vi "WildBugChilGru_V1.0.3.vi"() -> ()   [LabVIEW 2014]
uses:
  <vilib>/Utility/miscctls.llb/LVPointTypeDef.ctl
  <vilib>/Utility/xml.llb/Read From XML File(string).vi
  <vilib>/Utility/xml.llb/Write to XML File(string).vi
  <vilib>/gmath/NI_Gmath.lvlib
  <vilib>/Analysis/NI_AALBase.lvlib
  <vilib>/Analysis/NI_AALPro.lvlib
  <vilib>/Analysis/3filter.llb/IIR Filter (DBL).vi
  <vilib>/Instr/_visa.llb/VISA Configure Serial Port (Instr).vi
panel:
  in  "Registerkarte":T1(tab)
  in  "Zündung [Imp/U]":dbl=1.0
  in  "Übersetzung ermitteln aus":T2(ring)
  in  "Getriebe [1:]":dbl=5.343
  in  "Reifenumfang [m]":dbl=1.222
  in  "Dauer [s]":dbl=5.0
  in  "nKuWe/nRolle":dbl=10.0
  in  "Lufttemperatur [°C]":dbl=20.0
  in  "Luftfeuchtigkeit [%]":dbl=50.0
  in  "Luftdruck [mbar]":dbl=1013.0
  in  "Messung Klimadaten":bool=TRUE
  in  "Gleitender Mittelwert":u8=35
  in  "Differenzenquotient":u8=12
  in  "Polynom":u8=15
  in  "n vom Gas [1/min]":dbl=5000.0
  in  "Rollengeber [Inkr/U]":u16=200
  in  "Rollenumfang [m]":dbl=0.613
  in  "Rollenträgheit [kgm²]":dbl=0.402
  in  "Recalc":bool
  in  "Ende":bool
  out "Datenspeicher":T3={"Fahrzeugdaten"="", "date/time string"="", "Rolle [Inkr/U]"=0, "Rollenumfang [m]"=0.0, "Rollenträgheit [kgm²]"=0.0, "Zündung [Imp/U]"=0.0, "Getriebe [1:]"=0.0, "Reifenumfang [m] "=0.0, "element"=0.0, "Gl. Mittelwert"=0, "Differenzenquotient"=0, "Polynom"=0, "element"=0.0, "element"=0.0, "Lufttemperatur [°C]"=0.0, "Luftfeuchtigkeit [%]"=0.0, "Luftdruck [mbar]"=0.0, [], [], "Best Polynomial Fit"=[], [], "Übersetzung ermitteln aus"=0, "[s]"=0.0, "nmin [1/min]"=0.0, "nmax [1/min]"=0.0, "n vom Gas [1/min]"=0.0, [], [], "Boolesch"=FALSE, "Serielle Schnittstelle"="COM4", "nKuWe/nRolle"=10.0}
  out "COM-Fehlerrate":string="0 / 0,0%"
  in  "Konfiguration:":bool
  in  "Speichern":bool
  in  "Drucken":bool
  out "Pmax":string="0,0 PS"
  out "Ergebnis":string="0,0 PS bei 0 1/min   |   0,0 Nm bei 0 1/min   |   vmax: 2147483647 km/h\nDIN 70020 k =1,000 (20 °C, 50 %, 1013 mbar)\n20.11.2016 20:05 "
  in  "Fahrzeugdaten":string="Hier die Fahrzeugdaten eingeben"
  out "XY-Graph":cluster{dbl[], dbl[]}[](graph)
  out "Untersetzung\nermittelt":bool
  out "Untersetzung":dbl format="%#.2f"
  in  "Start":bool
  out "Füllstand Lesepuffer":u64(slide) scale=1.0..100.0
  out "Hinterrad\n[km/h]":dbl(knob) scale=0.0..150.0
  out "Welle\n[1/min]":cluster{dbl, dbl}(knob) scale=0.0..12000.0
  out "Lesepuffer":string="\n"
  in  "Serielle Schnittstelle":refnum<visa-resource-name>="COM4"
  out "Untersetzung-Graph":dbl(graph)=2.6802446808510636 caption="Untersetzung"
  # "1. n konstant halten\n2. START\n3. n weiter halten\n4. bei GO: Vollgas\n5. vom Gas gehen"
  # "Zündung\nRolle"
  # "Untersetzung aus:"
  # "Eingabe <> Messen"
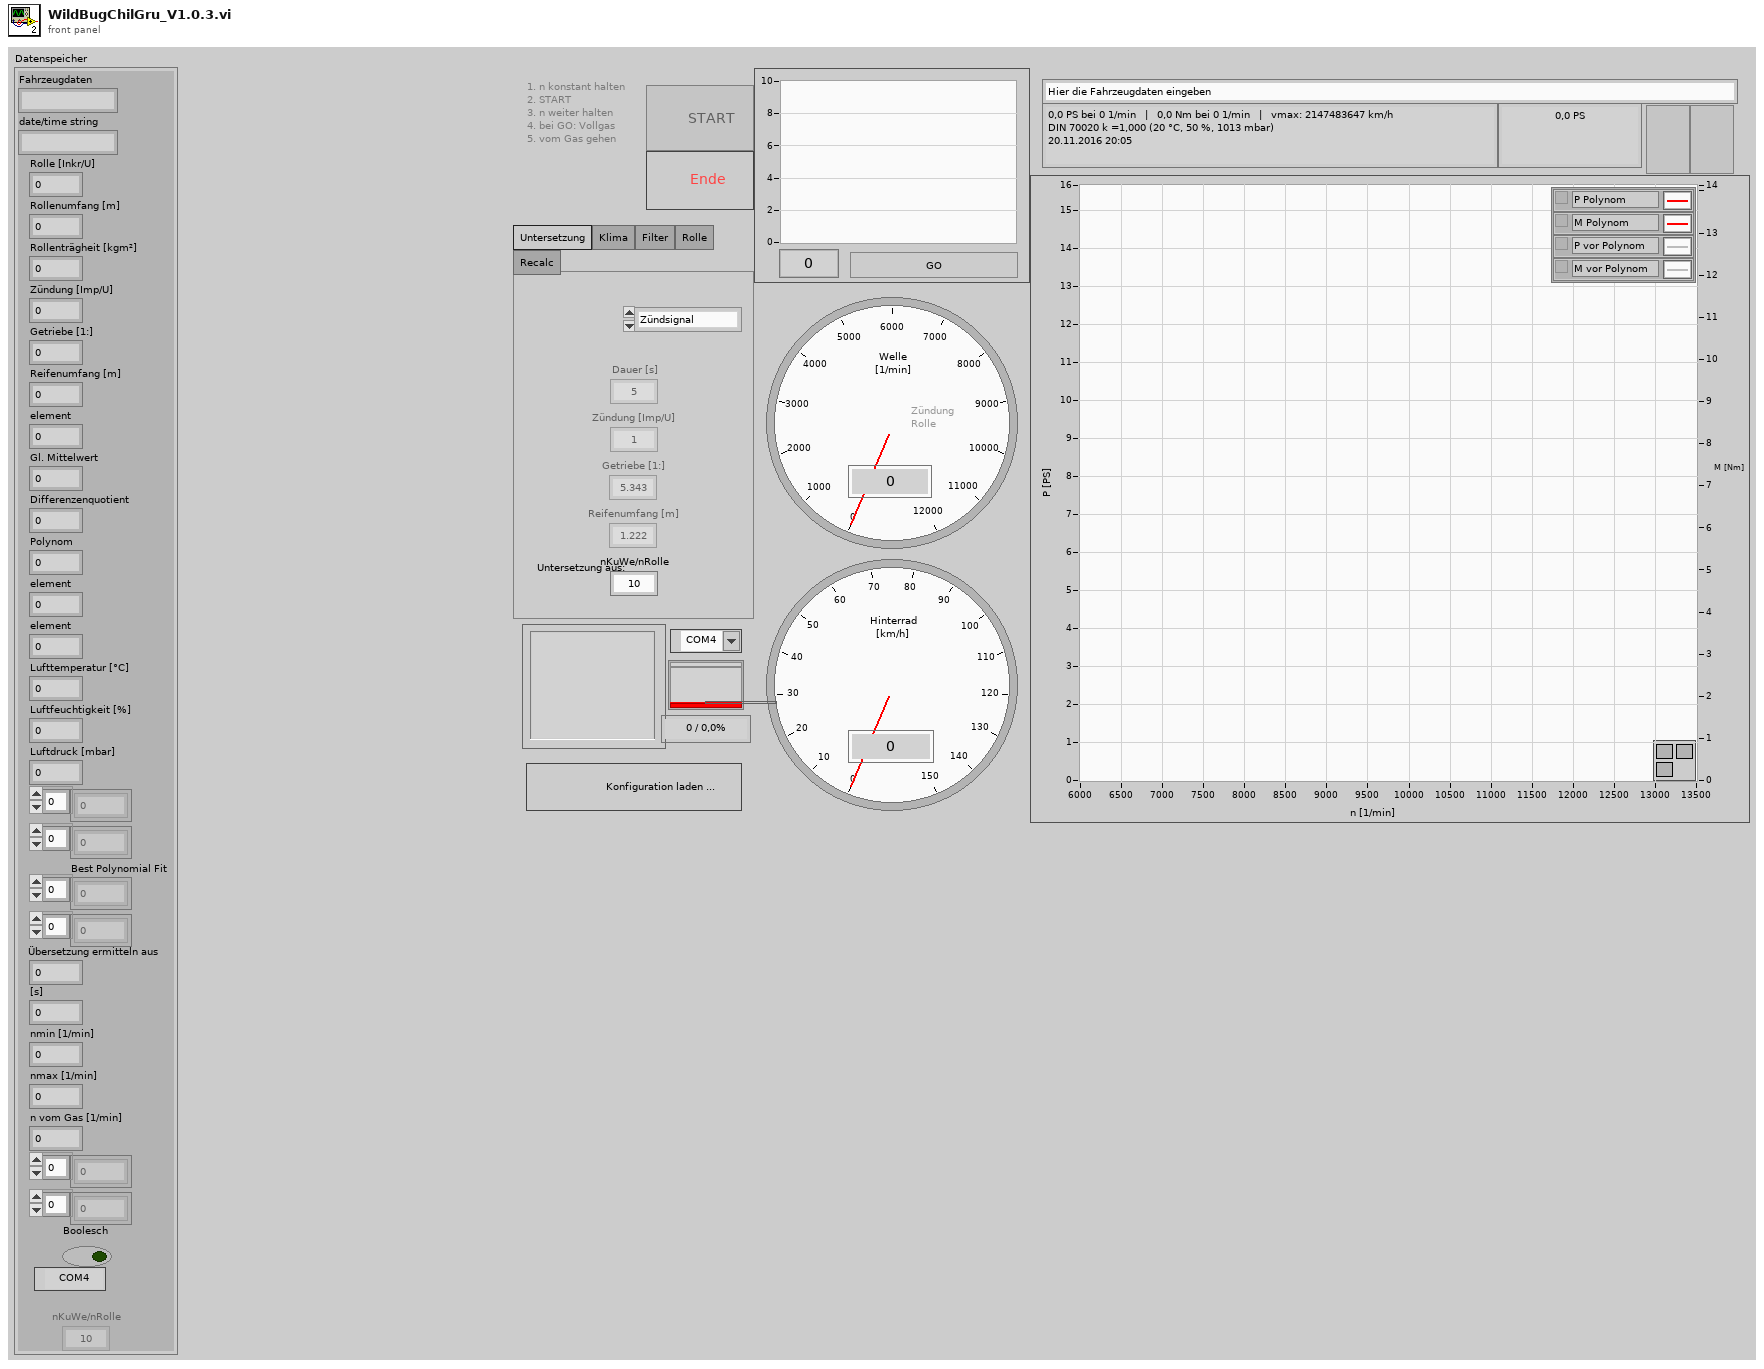
[diagram p1: front panel]
types:
  T1 = enum32{"Untersetzung", "Klima", "Filter", "Rolle", "Recalc"}
  T2 = enum8{"Zündsignal", "Getriebe & Reifen", "nKuWe / nRolle"}
  T3 = cluster{"Fahrzeugdaten":string, "date/time string":string, "Rolle [Inkr/U]":u16, "Rollenumfang [m]":dbl, "Rollenträgheit [kgm²]":dbl, "Zündung [Imp/U]":dbl, "Getriebe [1:]":dbl, "Reifenumfang [m] ":dbl, "element":dbl, "Gl. Mittelwert":u8, "Differenzenquotient":u8, "Polynom":u8, "element":dbl, "element":dbl, "Lufttemperatur [°C]":dbl, "Luftfeuchtigkeit [%]":dbl, "Luftdruck [mbar]":dbl, dbl[], dbl[], "Best Polynomial Fit":dbl[], dbl[], "Übersetzung ermitteln aus":u8, "[s]":dbl, "nmin [1/min]":dbl, "nmax [1/min]":dbl, "n vom Gas [1/min]":dbl, dbl[], i32[], "Boolesch":bool, "Serielle Schnittstelle":refnum<visa-resource-name>, "nKuWe/nRolle":dbl}
  T4 = enum16{"Kleinste Quadrate", "Kleinestes absolutes Reiduum", "Biquadrat"}
  T5 = enum8{"Enabled", "Disabled", "Disabled and Grayed Out"}
  T6 = cluster{"Fahrzeugdaten":string, "date/time string":string, "Rollengeber [Inkr/U]":u16, "Rollenumfang [m]":dbl, "Rollenträgheit [kgm²]":dbl, "Zündung [Imp/U]":dbl, "Getriebe [1:]":dbl, "Reifenumfang [m] ":dbl, "mean value":dbl, "Gleitender Mittelwert":u8, "Differenzenquotient":u8, "Polynom":u8, dbl, "element":dbl, "Lufttemperatur [°C]":dbl, "Luftfeuchtigkeit [%]":dbl, "Luftdruck [mbar]":dbl, dbl[], dbl[], "Best Polynomial Fit":dbl[], dbl[], "Übersetzung ermitteln aus":enum8{"Zündsignal", "Getriebe & Reifen", "nKuWe / nRolle"}, "Dauer [s]":dbl, dbl, dbl, "n vom Gas [1/min]":dbl, dbl[], i32[], "Messung Klimadaten":bool, "VISA resource name out":refnum<visa-resource-name>, "nKuWe/nRolle":dbl}
  T7 = cluster{"Fahrzeugdaten":string, "date/time string":string, "Rolle [Inkr/U]":u16, "Rollenumfang [m]":dbl, "Rollenträgheit [kgm²]":dbl, "Zündung [Imp/U]":dbl, "Getriebe [1:]":dbl, "Reifenumfang [m] ":dbl, "element":dbl, "Gl. Mittelwert":u8, "Differenzenquotient":u8, "Polynom":u8, "element":dbl, "element":dbl, "Lufttemperatur [°C]":dbl, "Luftfeuchtigkeit [%]":dbl, "Luftdruck [mbar]":dbl, dbl[], dbl[], "Best Polynomial Fit":dbl[], dbl[], "Übersetzung ermitteln aus":u8, "[s]":dbl, "nmin [1/min]":dbl, "nmax [1/min]":dbl, "n vom Gas [1/min]":dbl, dbl[], i32[], "Boolesch":bool, "Serielle Schnittstelle":refnum<visa-resource-name>, dbl}
  T8 = typedef "LVPointTypeDef.ctl" = cluster{"Horizontal":i16, "Vertical":i16}
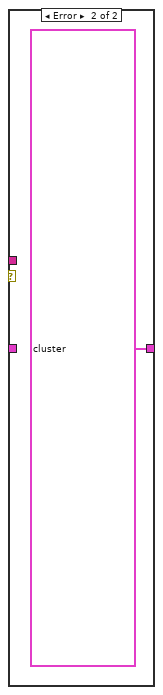
[diagram p2: hidden frame]
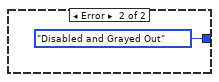
[diagram p3: hidden frame]
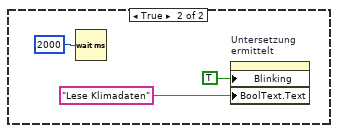
[diagram p5: hidden frame]
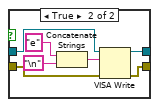
[diagram p6: hidden frame]
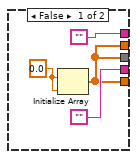
[diagram p8: hidden frame]
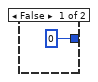
[diagram p9: hidden frame]
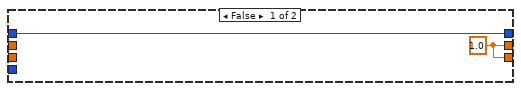
[diagram p11: hidden frame]
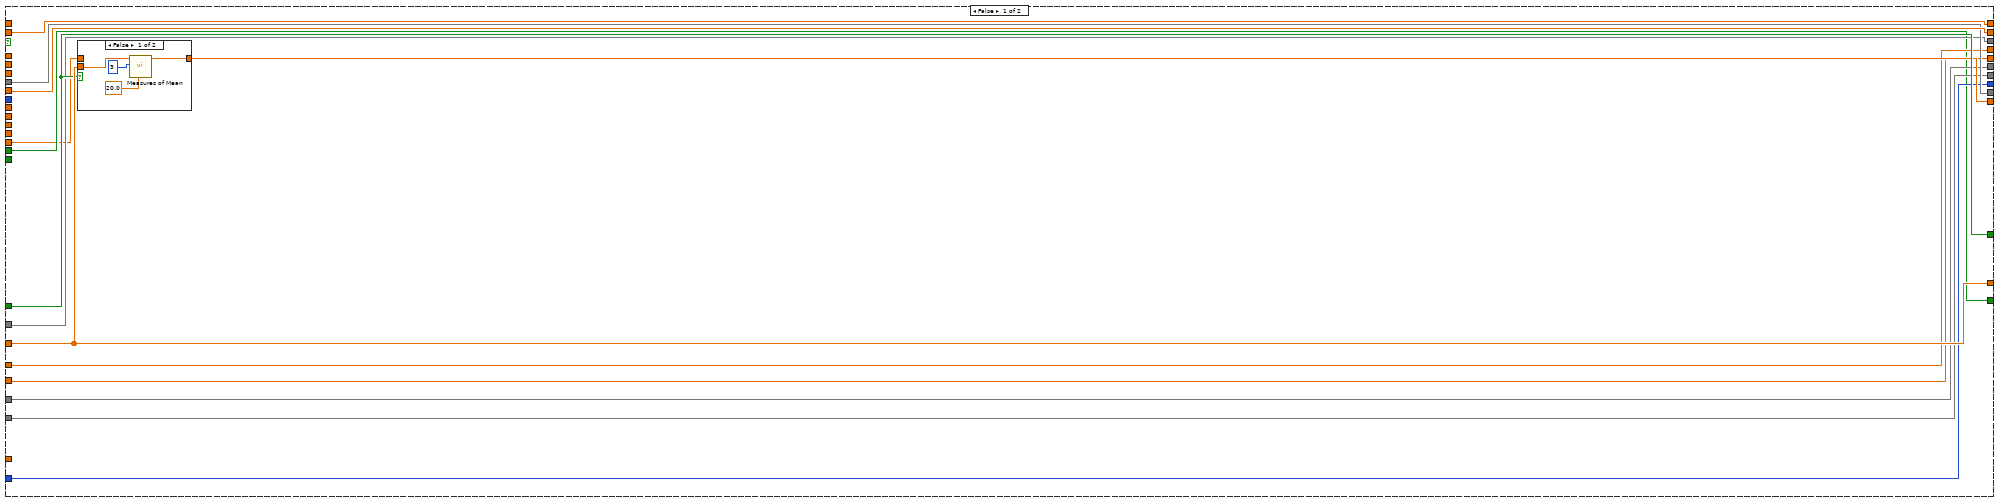
[diagram p12: hidden frame]
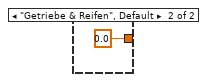
[diagram p16: hidden frame]
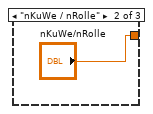
[diagram p18: hidden frame]
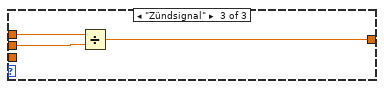
[diagram p19: hidden frame]
diagram:
  n1 = while {
    stop <- w1 stop-if-true
    n2 = local read "Start"() -> (w2:bool)
    n3 = case shown="True" w2 {
      frame False {
      }
      frame True {
        n4 = flat-sequence {
          tunnel: [w133] -> w118
          tunnel: [w132] -> w117
          tunnel: ["Messung Klimadaten"] -> w116
          tunnel: w118 -> [w146]
          tunnel: w117 -> [w145]
          tunnel: [0] -> w115
          tunnel: [1.0 ("element")] -> w114
          tunnel: [w143] -> w113
          tunnel: [w157] -> w112
          tunnel: [0] -> w111
          tunnel: [w143] -> w110
          tunnel: [-5] -> w109
          tunnel: [w154] -> w108
          tunnel: [w152] -> w107
          tunnel: [w151] -> w106
          tunnel: [0.0] -> w105
          tunnel: [w146] -> w104
          tunnel: [w145] -> w103
          tunnel: w116 -> [w144]
          tunnel: [w144] -> w102
          tunnel: w115 -> [w183]
          tunnel: [w183] -> w101
          tunnel: w114 -> [w182]
          tunnel: [w182] -> w100
          tunnel: w113 -> [w181]
          tunnel: [w181] -> w99
          tunnel: w112 -> [w180]
          tunnel: [w180] -> w98
          tunnel: w111 -> [w179]
          tunnel: [w179] -> w97
          tunnel: w110 -> [w178]
          tunnel: [w178] -> w96
          tunnel: w109 -> [w177]
          tunnel: [w177] -> w95
          tunnel: w108 -> [w176]
          tunnel: [w176] -> w94
          tunnel: w107 -> [w175]
          tunnel: [w175] -> w93
          tunnel: w106 -> [w174]
          tunnel: [w174] -> w92
          tunnel: w105 -> [w173]
          tunnel: [w173] -> w91
          tunnel: w104 -> [w172]
          tunnel: [w169] -> w90
          tunnel: w103 -> [w171]
          tunnel: [w170] -> w89
          tunnel: [w168] -> w88
          tunnel: w102 -> [w168]
          tunnel: w101 -> [w207]
          tunnel: [w207] -> w87
          tunnel: w100 -> [w206]
          tunnel: [w206] -> w86
          tunnel: w99 -> [w205]
          tunnel: [w205] -> w85
          tunnel: w98 -> [w204]
          tunnel: [w204] -> w84
          tunnel: w97 -> [w203]
          tunnel: [w203] -> w83
          tunnel: w96 -> [w202]
          tunnel: [w202] -> w82
          tunnel: w95 -> [w201]
          tunnel: [w201] -> w81
          tunnel: w94 -> [w200]
          tunnel: [w200] -> w80
          tunnel: w93 -> [w199]
          tunnel: [w199] -> w79
          tunnel: w92 -> [w198]
          tunnel: [w198] -> w78
          tunnel: w91 -> [w197]
          tunnel: [w197] -> w77
          tunnel: w90 -> [w196]
          tunnel: [w196] -> w76
          tunnel: w89 -> [w195]
          tunnel: [w195] -> w75
          tunnel: w88 -> [w193]
          tunnel: [w193] -> w74
          tunnel: w87 -> [w223]
          tunnel: [w223] -> w73
          tunnel: w86 -> [w222]
          tunnel: [w222] -> w72
          tunnel: w85 -> [w221]
          tunnel: [w221] -> w71
          tunnel: w84 -> [w220]
          tunnel: [w220] -> w70
          tunnel: w83 -> [w219]
          tunnel: [w219] -> w69
          tunnel: w82 -> [w218]
          tunnel: [w218] -> w68
          tunnel: w81 -> [w217]
          tunnel: [w217] -> w67
          tunnel: w80 -> [w216]
          tunnel: [w216] -> w66
          tunnel: w79 -> [w215]
          tunnel: [w215] -> w65
          tunnel: w78 -> [w214]
          tunnel: [w214] -> w64
          tunnel: w77 -> [w213]
          tunnel: [w213] -> w63
          tunnel: w76 -> [w212]
          tunnel: [w211] -> w62
          tunnel: w75 -> [w209]
          tunnel: [w210] -> w61
          tunnel: w74 -> [w208]
          tunnel: w73 -> [w297]
          tunnel: w72 -> [w296]
          tunnel: w71 -> [w295]
          tunnel: w70 -> [w294]
          tunnel: w69 -> [w293]
          tunnel: w68 -> [w292]
          tunnel: w67 -> [w291]
          tunnel: w66 -> [w290]
          tunnel: w65 -> [w289]
          tunnel: w64 -> [w288]
          tunnel: w63 -> [w287]
          tunnel: w62 -> [w252]
          tunnel: [w297] -> w60
          tunnel: [w296] -> w59
          tunnel: [w295] -> w58
          tunnel: [w294] -> w57
          tunnel: [w293] -> w56
          tunnel: [w292] -> w55
          tunnel: [w291] -> w54
          tunnel: [w290] -> w53
          tunnel: [w289] -> w52
          tunnel: [w288] -> w51
          tunnel: [w287] -> w50
          tunnel: [w252] -> w49
          tunnel: [w251] -> w48
          tunnel: [w286] -> w47
          tunnel: [w285] -> w46
          tunnel: [w284] -> w45
          tunnel: ["Gleitender Mittelwert"] -> w44
          tunnel: w61 -> [w251]
          tunnel: [w306] -> w10
          tunnel: [w307] -> w11
          tunnel: [w308] -> w12
          tunnel: [w309] -> w13
          tunnel: [w300] -> w8
          tunnel: [w299] -> w9
          tunnel: [w310] -> w14
          tunnel: [w311] -> w15
          tunnel: [w312] -> w17
          tunnel: [w313] -> w19
          tunnel: [w314] -> w20
          tunnel: [w315] -> w21
          tunnel: [w316] -> w38
          tunnel: [w317] -> w40
          tunnel: [w318] -> w41
          tunnel: [w319] -> w42
          tunnel: [w320] -> w43
          tunnel: w60 -> [w320]
          tunnel: w59 -> [w319]
          tunnel: w58 -> [w318]
          tunnel: w57 -> [w317]
          tunnel: w56 -> [w316]
          tunnel: w55 -> [w315]
          tunnel: w54 -> [w314]
          tunnel: w53 -> [w313]
          tunnel: w52 -> [w312]
          tunnel: w51 -> [w311]
          tunnel: w50 -> [w310]
          tunnel: w49 -> [w302]
          tunnel: w48 -> [w301]
          tunnel: w47 -> [w309]
          tunnel: w46 -> [w308]
          tunnel: w45 -> [w307]
          tunnel: w44 -> [w306]
          frame #0 {
            w138 = u16 0 items=["None", "XON/XOFF", "RTS/CTS", "XON/XOFF & RTS/CTS", "DTR/DSR", "XON/XOFF & DTR/DSR"] ("flow control (0:none)")
            w139 = u16 10 items=["1.0"=10, "1.5"=15, "2.0"=20] ("stop bits (10: 1 bit)")
            w131 = FALSE  # Enable Termination Char (T)
            w134 = u32 10000  # timeout (10sec)
            n5 = call-poly "VISA Configure Serial Port"("VISA resource name"="Serielle Schnittstelle", "timeout (10sec)"=w134, "Enable Termination\nChar (T)"=w131, "baud rate (9600)"=u32 115200 ("baudrate (250000)"), "data bits (8)"=u16 8, "parity (0:none)"=enum16{"None", "Odd", "Even", "Mark", "Space"}."None", "stop bits (10: 1 bit)"=w139, "flow control (0:none)"=w138) -> ("VISA resource name out"=w136:refnum<visa-resource-name>, "error out"=w135:errorcluster)  [unwired: 6 in]
            n6 = VISA Clear(VISA resource name=w136, error in (no error)=w135) -> (VISA resource name out=w133:refnum<visa-resource-name>, error out=w132:errorcluster)
          }
          frame #1 {
            w147 = T5."Disabled and Grayed Out" ("Deaktiviert")
            w150 = 0.0  # Graphen löschen
            w153 = 0
            w158 = 0.0
            w143 = FALSE
            w151 = ""
            n7 = case shown="False" w144 {
              frame False {
                n8 = property on="Untersetzung\nermittelt" class="Bool. (strikt)"("Blinking"=TRUE ("Blinkend"), "BoolText.Text"="Initialisiere" ("Beschriftung.Text")) -> ()  [unwired: 2 in, 2 out]
              }
              frame True {
                n9 = Wait (ms)(milliseconds to wait=u32 2000 ("Zu wartende ms")) -> ()  [unwired: 1 out]
                n10 = property on="Untersetzung\nermittelt" class="Bool. (strikt)"("Blinking"=TRUE ("Blinkend"), "BoolText.Text"="Lese Klimadaten" ("Beschriftung.Text")) -> ()  [unwired: 2 in, 2 out]
              }
            }
            n11 = Build Array(w150) -> (w149:dbl[])
            n12 = property on="Drucken" class="Bool. (strikt)"("DisabledEnum"=w147) -> ()  [unwired: 2 in, 2 out]
            n13 = property on="Übersetzung ermitteln aus" class="Enum (strikt)"("DisabledEnum"=w147) -> ()  [unwired: 2 in, 2 out]
            n14 = property on="Konfiguration:" class="Bool. (strikt)"("DisabledEnum"=w147) -> ()  [unwired: 2 in, 2 out]
            n15 = property on="Ende" class="Bool. (strikt)"("DisabledEnum"=w147) -> ()  [unwired: 2 in, 2 out]
            n16 = property on="Speichern" class="Bool. (strikt)"("DisabledEnum"=w147) -> ()  [unwired: 2 in, 2 out]
            n17 = property on="Untersetzung-Graph" class="SVDiagr (strikt)"("History Data"=w149) -> ()  [unwired: 2 in, 2 out]
            n18 = local write "Pmax"(w151) -> ()
            n19 = local write "COM-Fehlerrate"(w151) -> ()
            n20 = local write "Ergebnis"(w151) -> ()
            n21 = Initialize Array(w158, w158) -> (w157:dbl[])
            n22 = Initialize Array(0.0 ("y"), 0) -> (w154:dbl[])
            n23 = Initialize Array(w153, w153) -> (w152:i32[])
          }
          frame #2 {
            n24 = case shown="False" w168 {
              tunnel: w172 -> [w185 w189]
              tunnel: w171 -> [w184 w188]
              tunnel: [w184 w187] -> w170
              tunnel: [w185 w186] -> w169
              frame False {
              }
              frame True {
                n25 = Concatenate Strings("e" ("String"), "\n") -> (w192:string)
                n26 = VISA Write(VISA resource name=w189, write buffer=w192, error in (no error)=w188) -> (VISA resource name out=w186:refnum<visa-resource-name>, error out=w187:errorcluster)  [unwired: 1 out]
              }
            }
          }
          frame #3 {
            n27 = Wait (ms)(milliseconds to wait=u32 500 ("Zu wartende ms")) -> ()  [unwired: 1 out]
          }
          frame #4 {
            n28 = case shown="True" w208 {
              tunnel: w212 -> [w225 w246]
              tunnel: [w225 w245] -> w211
              tunnel: [w224 w244] -> w210
              tunnel: w209 -> [w224 w243]
              frame False {
              }
              frame True {
                w228 = ";" ("Regulärer Ausdruck")
                n29 = property class="Instr"(reference=w246, error in=w243) -> (reference out=w249:refnum<visa-resource-name>, error out=w248:errorcluster, "Serial Settings:Number of Bytes at Serial Port"=w247:u32)
                n30 = VISA Read(VISA resource name=w249, byte count=w247, error in (no error)=w248) -> (VISA resource name out=w245:refnum<visa-resource-name>, read buffer=w240:string, error out=w244:errorcluster)  [unwired: 1 out]
                n31 = Search and Replace String(replace all?=TRUE ("Alle ersetzen? (F)"), input string=w240, search string="." ("Such-String"), replace string="," ("Ersetzungs-String (\"\")")) -> (result string=w233:string)  [unwired: 4 in, 3 out]
                n32 = Match Pattern(string=w233, regular expression=w228) -> (before substring=w231:string, after substring=w232:string)  [unwired: 1 in, 2 out]
                n33 = Match Pattern(string=w232, regular expression=w228) -> (before substring=w230:string, after substring=w229:string)  [unwired: 1 in, 2 out]
                n34 = Fract/Exp String To Number(string=w231, offset=0 ("Offset")) -> (number=w239:dbl)  [unwired: 2 in, 1 out]
                n35 = local write "Lufttemperatur [°C]"(w239) -> ()
                n36 = Fract/Exp String To Number(string=w230) -> (number=w236:dbl)  [unwired: 3 in, 1 out]
                n37 = Match Pattern(string=w229, regular expression=w228) -> (before substring=w227:string)  [unwired: 1 in, 3 out]
                n38 = Fract/Exp String To Number(string=w227) -> (number=w238:dbl)  [unwired: 3 in, 1 out]
                n39 = Divide(x=w236, y=100.0 ("x")) -> (x/y=w237:dbl)
                n40 = local write "Luftdruck [mbar]"(w237) -> ()
                n41 = local write "Luftfeuchtigkeit [%]"(w238) -> ()
              }
            }
          }
          frame #5 {
            n42 = Wait (ms)(milliseconds to wait=u32 2000 ("Zu wartende ms")) -> ()  [unwired: 1 out]
            n43 = Add(x="Lufttemperatur [°C]", y=273.15) -> (x+y=w267:dbl)
            n44 = Divide ("M_Welle [Nm]")(x=300.0, y=w267) -> (x/y=w270:dbl)
            n45 = Multiply(x="Luftfeuchtigkeit [%]", y=0.01) -> (x*y=w281:dbl)
            n46 = Divide ("M_Welle [Nm]")(x=w267, y=293.15) -> (x/y=w265:dbl)
            n47 = Multiply(x=w281, y=240800000000.0) -> (x*y=w255:dbl)
            n48 = Power Of X(1:w270, 2:5.0) -> (0:w268:dbl)
            n49 = Multiply(x=w255, y=w268) -> (x*y=w275:dbl)
            n50 = Multiply(x=w270, y=-22.644) -> (x*y=w276:dbl)
            n51 = Power Of X(1:w265, 2:0.5) -> (0:w262:dbl)
            n52 = Exponential(1:w276) -> (0:w274:dbl)
            n53 = Multiply(x=w275, y=w274) -> (x*y=w273:dbl)
            n54 = Subtract "p_Trocken [mbar]"(x="Luftdruck [mbar]", y=w273) -> (x-y=w271:dbl)
            n55 = Divide ("M_Welle [Nm]")(x=1013.0, y=w271) -> (x/y=w263:dbl)
            n56 = Multiply "Korrekturfaktor DIN 70020"(x=w263, y=w262) -> (x*y=w286:dbl)
            n57 = Divide(x="Gleitender Mittelwert", y=2) -> (x/y=w259:dbl)
            n58 = Round Toward -Infinity(1:w259) -> (0:w258:dbl)
            n59 = call <vilib>:"Smoothing Filter Coefficients.vi"("shape"=1, "half-width"=w258, "type"=0) -> ("forward coefficients"=w284:dbl[], "reverse coefficients"=w285:dbl[])  [unwired: 6 in, 1 out]
          }
          frame #6 {
            n60 = Concatenate Strings("m" ("String"), "\n") -> (w305:string)
            n61 = property on="Untersetzung\nermittelt" class="Bool. (strikt)"("Blinking"=FALSE ("Blinkend")) -> ()  [unwired: 2 in, 2 out]
            n62 = VISA Write(VISA resource name=w302, write buffer=w305, error in (no error)=w301) -> (VISA resource name out=w299:refnum<visa-resource-name>, error out=w300:errorcluster)  [unwired: 1 out]
          }
        }
        n63 = while {
          tunnel: w9 -> [w454]
          tunnel: w8 -> [w453]
          shift-right: [w524] -> _
          shift-left: w15 -> [w469]
          shift-right: [w519] -> _
          shift-left: w14 -> [w523]
          shift-right: [w518] -> _
          shift-left: w14 -> [w522]
          shift-right: [w473] -> _
          shift-left: w14 -> [w521]
          shift-right: [w500] -> _
          shift-left: w43 -> [w520]
          shift-right: [w461] -> w26
          shift-left: w42 -> [_]
          shift-right: [w479] -> w30
          shift-left: w14 -> [w501]
          shift-right: [w511] -> w28
          shift-left: w14 -> [w475]
          shift-right: [w474] -> _
          shift-left: w19 -> [w515]
          shift-right: [w512] -> _
          shift-left: w41 -> [w489]
          shift-right: [w455] -> _
          shift-left: w40 -> [_]
          shift-right: [w460] -> _
          shift-left: w40 -> [_]
          shift-right: [w510] -> w29
          shift-left: w40 -> [w508]
          shift-right: [w509] -> _
          shift-left: w40 -> [w507]
          shift-right: [w495] -> w37
          shift-left: w19 -> [w506]
          shift-right: [w499] -> _
          shift-left: w19 -> [w504]
          shift-right: [w498] -> w33
          shift-left: w19 -> [w505]
          shift-right: [w497] -> w36
          shift-left: w19 -> [w503]
          shift-right: [w496] -> w35
          shift-left: w19 -> [w502]
          tunnel: [w494] -> w39
          shift-right: [w490] -> w34
          shift-left: w38 -> [w492]
          tunnel: [w493] -> w5
          tunnel: ["n vom Gas [1/min]"] -> w32
          tunnel: ["Rollenumfang [m]"] -> w31
          tunnel: ["Rollenumfang [m]"] -> w25
          shift-right: [w486] -> _
          shift-left: w21 -> [w452]
          shift-right: [w480] -> _
          shift-left: w20 -> [w485]
          shift-right: [w481] -> _
          shift-left: w14 -> [w484]
          shift-right: [w482] -> _
          shift-left: w14 -> [w483]
          shift-right: [w478] -> w18
          shift-left: w19 -> [w477]
          shift-right: [w472] -> _
          shift-left: _ -> [w471]
          shift-right: [w476] -> w16
          shift-left: w17 -> [w470]
          tunnel: [w468] -> w6
          tunnel: w13 -> [w461]
          tunnel: w12 -> [w455]
          tunnel: w11 -> [w460]
          tunnel: w10 -> [w459]
          stop <- w494 stop-if-true
          n64 = property class="Instr"(reference=w454, error in=w453) -> (reference out=w464:refnum<visa-resource-name>, error out=w463:errorcluster, "Serial Settings:Number of Bytes at Serial Port"=w466:u32)
          n65 = Greater?(x=w466, y=u32 1 ("min. Bytes")) -> (0:w462:bool)
          n66 = case shown="True" w462 {
            tunnel: w466 -> [_ w526]
            tunnel: [u32 0 ("Bytes at Port") w526] -> w465
            frame False {
            }
            frame True {
            }
          }
          n67 = case shown="1.." w465 {
            selector: w465 -> [_ w779]
            tunnel: [w729 w773] -> w493
            tunnel: [w728 w774] -> w468
            tunnel: [w733 w775] -> w518
            tunnel: [w734 w772] -> w519
            tunnel: w469 -> [w735 w770]
            tunnel: [w735 w768] -> w524
            tunnel: w523 -> [w734 w760]
            tunnel: w522 -> [w733 w759]
            tunnel: [w730 w758] -> w473
            tunnel: w521 -> [w730 w757]
            tunnel: w520 -> [w732 _]
            tunnel: [w732 w740] -> w500
            tunnel: [w731 w746] -> w472
            tunnel: w471 -> [w731 w745]
            tunnel: w464 -> [w728 w737]
            tunnel: w463 -> [w729 w736]
            frame 0, Default {
              # "No data in from serial port - Nothing to do."
            }
            frame 1.. {
              # "Hz Drum"
              n68 = VISA Read(VISA resource name=w737, byte count=w779, error in (no error)=w736) -> (VISA resource name out=w774:refnum<visa-resource-name>, read buffer=w771:string, error out=w773:errorcluster)  [unwired: 1 out]
              n69 = Concatenate Strings(w770, w771) -> (w742:string)
              "Lesepuffer" <- w742
              n70 = Spreadsheet String To Array(delimiter (Tab)="\n" ("regular expression"), format string="%s" ("regular expression"), spreadsheet string=w742, array type (2D Dbl)=string[] [] ("Array 2")) -> (array=w751:string[])
              n71 = Match Pattern(string=w742, regular expression="[\\n]") -> (before substring=w749:string, after substring=w769:string, offset past match=w783:i32)  [unwired: 1 in, 1 out]
              n72 = Array Size(array=w751) -> (size(s)=w755:i32)
              n73 = Match Pattern(string=w749, regular expression="[;]") -> (before substring=w747:string, after substring=w748:string, offset past match=w744:i32)  [unwired: 1 in, 1 out]
              n74 = Subtract "aktuelle Zeilenanzahl"(x=w755, y=1) -> (x-y=w740:i32)
              n75 = property on="Füllstand Lesepuffer" class="Schieber (strikt)"() -> ("Scale.Maximum"=w739:dbl)  [unwired: 2 in, 2 out]
              n76 = Match Pattern(string=w748, regular expression="[;]") -> (before substring=w778:string, after substring=w781:string, offset past match=w766:i32)  [unwired: 1 in, 1 out]
              n77 = Match Pattern(string=w781, regular expression="[;]") -> (before substring=w777:string, after substring=w776:string, offset past match=w764:i32)  [unwired: 1 in, 1 out]
              n78 = Greater Or Equal To 0?(x=w744) -> (x >= 0?=w743:bool)
              n79 = Greater?(x=w740, y=w739) -> (0:w741:bool)
              n80 = Greater Or Equal To 0?(x=w764) -> (x >= 0?=w763:bool)
              n81 = Greater Or Equal To 0?(x=w766) -> (x >= 0?=w765:bool)
              n82 = Greater Or Equal To 0?(x=w783) -> (x >= 0?=w767:bool)
              n83 = Select(t=w740, s=w741, f=w739) -> (s? t:f=w738:dbl)
              n84 = Build Array(w767, w765, w743, w763) -> (w762:bool[])
              n85 = property on="Füllstand Lesepuffer" class="Schieber (strikt)"("Scale.Maximum"=w738) -> ()  [unwired: 2 in, 2 out]
              n86 = And Array Elements(Boolean array=w762) -> (logical AND=w761:bool)
              n87 = case shown="True" w761 {
                tunnel: w778 -> [_ w794]
                tunnel: w777 -> [_ w799]
                tunnel: w776 -> [_ w798]
                tunnel: [w787 w797] -> w775
                tunnel: [w788 w796] -> w772
                tunnel: w769 -> [_ w795]
                tunnel: [w789 w795] -> w768
                tunnel: w742 -> [w789 _]
                tunnel: w760 -> [w788 _]
                tunnel: w759 -> [w787 _]
                tunnel: [w786 w793] -> w758
                tunnel: w757 -> [w786 _]
                tunnel: w747 -> [_ w792]
                tunnel: [w785 w790] -> w746
                tunnel: w745 -> [w785 _]
                frame False {
                }
                frame True {
                  # "Cyclecounter"
                  # "Hz ComLevel"
                  # "ComLevel\nLevel 10 =   6Hz \nLevel 5 =   12Hz \nLevel 4 =   15Hz\nLevel 3 =   20Hz\nLevel 2 =   33Hz\nLevel 1 =   62Hz"
                  # "Hz Drum"
                  # "Hz Engine"
                  # "t4m"
                  n88 = Fract/Exp String To Number(string=w792) -> (number=w791:dbl)  [unwired: 3 in, 1 out]
                  n89 = Fract/Exp String To Number(string=w798) -> (number=w797:dbl)  [unwired: 3 in, 1 out]
                  n90 = Fract/Exp String To Number(string=w794) -> (number=w793:dbl)  [unwired: 3 in, 1 out]
                  n91 = To Long Integer(number=w791) -> (32bit integer=w790:i32)
                  n92 = Fract/Exp String To Number(string=w799) -> (number=w796:dbl)  [unwired: 3 in, 1 out]
                }
              }
            }
          }
          "Füllstand Lesepuffer" <- w500
          n93 = Not Equal?(x=w471, y=w472) -> (x != y?=w456:bool)
          n94 = case shown="True" w456 {
            tunnel: w485 -> [w530 w541]
            tunnel: [w530 w553] -> w480
            tunnel: w484 -> [w529 w552]
            tunnel: [w529 w538] -> w481
            tunnel: w483 -> [w528 w551]
            tunnel: [w528 w539] -> w482
            tunnel: w472 -> [_ w537]
            tunnel: w470 -> [w527 w536]
            tunnel: [w527 w540] -> w476
            frame False {
            }
            frame True {
              n95 = Build Array (concatenate)(w536, w537) -> (w540:i32[])
              n96 = Greater Or Equal To 0?(x=w541) -> (x >= 0?=w542:bool)
              n97 = case shown="True" w542 {
                tunnel: [w554 w565] -> w538
                tunnel: [w554 w566] -> w539
                tunnel: [w555 w557] -> w553
                tunnel: w552 -> [_ w559]
                tunnel: w551 -> [_ w567]
                tunnel: w537 -> [w555 w556]
                tunnel: w541 -> [_ w557]
                frame False {
                  w554 = 1.0
                }
                frame True {
                  w563 = 65536.0
                  n98 = Add(x=w557, y=w559) -> (x+y=w558:dbl)
                  n99 = Increment(x=w567) -> (x+1=w566:dbl)
                  n100 = Divide(x=w558, y=w563) -> (x/y=w568:dbl)
                  n101 = Round Toward -Infinity(1:w568) -> (0:w564:dbl)
                  n102 = Multiply(x=w564, y=w563) -> (x*y=w562:dbl)
                  n103 = Add(x=w562, y=w556) -> (x+y=w561:dbl)
                  n104 = Increment(x=w561) -> (x+1=w560:dbl)
                  n105 = Subtract(x=w560, y=w557) -> (x-y=w565:dbl)
                }
              }
              n106 = Subtract(x=w538, y=w539) -> (x-y=w533:dbl)
              n107 = Decrement(x=w533) -> (x-1=w532:dbl)
              n108 = Max & Min(x=0, y=w532) -> (max(x,y)=w531:dbl)  [unwired: 1 out]
              n109 = Divide(x=w531, y=w538) -> (x/y=w545:dbl)
              n110 = Greater Than 0?(x=w531) -> (x > 0?=w535:bool)
              n111 = Select(t=u32 16711680, s=w535, f=u32 0) -> (s? t:f=w546:u32)
              n112 = Multiply(x=w545, y=100.0) -> (x*y=w543:dbl)
              n113 = Format Into String(format string="%d / %.1f%%" ("Format-String"), w531, w543) -> (resulting string=→"COM-Fehlerrate":string)  [unwired: 2 in, 1 out]
              n114 = property on="COM-Fehlerrate" class="Str"("Text.TextColor"=w546) -> ()  [unwired: 2 in, 2 out]
            }
          }
          n115 = case "Case-Struktur" shown="True" w456 {
            tunnel: w519 -> [w709 w720]
            tunnel: w518 -> [w708 w719]
            tunnel: [w709 w718] -> w517
            tunnel: [w708 w717] -> w516
            tunnel: w473 -> [_ w711]
            tunnel: w501 -> [w707 _]
            tunnel: [w707 w710] -> w479
            tunnel: w475 -> [_ w716]
            tunnel: "Rollenumfang [m]" -> [_ w715]
            frame False {
            }
            frame True {
              w727 = 60.0 ("y")
              n116 = Reciprocal "Abtastzeit [s]"(x=w711) -> (1/x=w710:dbl)
              n117 = Divide "R [1/s]"(x=w719, y="Rollengeber [Inkr/U]") -> (x/y=w726:dbl)
              n118 = Divide(x=w720, y="Zündung [Imp/U]") -> (x/y=w723:dbl)
              n119 = Multiply "nZ gemessen [1/min]"(x=w723, y=w727) -> (x*y=w718:dbl)
              n120 = Multiply "nR [1/min]"(x=w727, y=w726) -> (x*y=w717:dbl)
              n121 = Multiply "nZ berechnet [1/min]"(x=w717, y=w716) -> (x*y=w725:dbl)
              n122 = Multiply "[m/min]"(x=w717, y=w715) -> (x*y=w721:dbl)
              n123 = Multiply "[km/h]"(x=w721, y=0.06) -> (x*y=→"Hinterrad\n[km/h]":dbl)
              n124 = Bundle(w718, w725) -> (→"Welle\n[1/min]":cluster{dbl, dbl})  [unwired: 1 in]
            }
          }
          n125 = case shown="True" w456 {
            tunnel: w517 -> [_ w638]
            tunnel: w516 -> [_ w637]
            tunnel: "Rollenumfang [m]" -> [_ w641]
            tunnel: [w580 w607] -> w511
            tunnel: w475 -> [w569 w607]
            tunnel: w489 -> [w581 w645]
            tunnel: w515 -> [w582 w644]
            tunnel: [w581 w598] -> w512
            tunnel: [w582 w643] -> w474
            tunnel: w455 -> [_ w640]
            tunnel: w460 -> [_ w639]
            tunnel: [w579 w593] -> w510
            tunnel: [w578 w591] -> w509
            tunnel: w508 -> [w579 w636]
            tunnel: w507 -> [w578 _]
            tunnel: w459 -> [_ w589]
            tunnel: [w577 w613] -> w495
            tunnel: w506 -> [w577 _]
            tunnel: [w576 w628] -> w499
            tunnel: w504 -> [w576 _]
            tunnel: w501 -> [_ w626]
            tunnel: [w575 w614] -> w498
            tunnel: w505 -> [w575 _]
            tunnel: [w574 w630] -> w497
            tunnel: w503 -> [w574 _]
            tunnel: [w573 w629] -> w496
            tunnel: w502 -> [w573 _]
            tunnel: w461 -> [_ w618]
            tunnel: w492 -> [w572 w612]
            tunnel: "n vom Gas [1/min]" -> [_ w600]
            tunnel: [w572 w611] -> w490
            tunnel: w489 -> [_ w610]
            tunnel: w452 -> [w571 w606]
            tunnel: [w571 w605] -> w486
            tunnel: w479 -> [_ w604]
            tunnel: [w570 w603] -> w478
            tunnel: w477 -> [w570 w602]
            frame False {
              n126 = case shown="False" w581 {
                tunnel: w582 -> [w586 _]
                tunnel: [w585 w587] -> w580
                tunnel: w569 -> [_ w587]
                frame False {
                  n127 = call <vilib>:"Measures of Mean.vi"("percent (trim)"=20.0, "type"=3, "x array"=w586) -> ("mean value"=w585:dbl)  [unwired: 7 in, 1 out]
                }
                frame True {
                }
              }
            }
            frame True {
              w621 = 0.00135962  # [W] in [PS]
              w632 = 0.10471975511965978  # 2*Pi/60
              n128 = Build Array (concatenate) "akt. dT in Array einfügen"(w602, w604) -> (w603:dbl[])
              n129 = Build Array (concatenate) "akt. Rollendrehzahl\nin Array einfügen"(w636, w637) -> (w593:dbl[])
              n130 = local read "Übersetzung ermitteln aus"() -> (w588:T2)
              n131 = Index Array(array=w593, index=1 ("Index")) -> (element=w596:dbl)
              n132 = case shown="\"Getriebe & Reifen\"" w588 {
                tunnel: w638 -> [_ _ w706]
                tunnel: w637 -> [_ _ w705]
                tunnel: [w701 "nKuWe/nRolle" w704] -> w642
                tunnel: w641 -> [w702 _ _]
                frame "Getriebe & Reifen" {
                  n133 = Divide(x=w702, y="Reifenumfang [m]") -> (x/y=w700:dbl)
                  n134 = Multiply(x=w700, y="Getriebe [1:]") -> (x*y=w701:dbl)
                }
                frame "nKuWe / nRolle" {
                }
                frame "Zündsignal" {
                  n135 = Divide(x=w706, y=w705) -> (x/y=w704:dbl)
                }
              }
              n136 = Initialize Array(w596, w589) -> (w595:dbl[])
              n137 = Insert Into Array(array=w593, index=0 ("Index"), new element=w595) -> (w592:dbl[])
              n138 = call-poly <vilib>:"IIR Filter.vi"("Forward Coefficients"=w639, "Reverse Coefficients"=w640, "X"=w592) -> ("Filtered X"=w590:dbl[])  [unwired: 1 in, 1 out]
              n139 = Array Subset(array=w590, index=w589) -> (w591:dbl[])  [unwired: 1 in]
              n140 = Multiply(x=2.0, y=w626) -> (x*y=w625:dbl)
              n141 = case shown="False" w645 {
                selector: w645 -> [_ w697]
                tunnel: w642 -> [w686 _]
                tunnel: w644 -> [w688 w696]
                tunnel: [w682 w697] -> w635
                tunnel: [w687 w696] -> w643
                tunnel: w606 -> [w685 w695]
                tunnel: [w682 w695] -> w605
                tunnel: w588 -> [w683 _]
                frame False {
                  n142 = Build Array (concatenate)(w688, w686) -> (w687:dbl[])
                  n143 = case shown="\"Zündsignal\"" w683 {
                    tunnel: ["Dauer [s]" 0.0 ("Dauer [s]")] -> w684
                    frame "Zündsignal" {
                      n144 = property on="Untersetzung\nermittelt" class="Bool. (strikt)"("Blinking"=TRUE ("Blinkend"), "BoolText.Text"="Ermittle Übersetzung" ("Boolescher Text.Text")) -> ()  [unwired: 2 in, 2 out]
                    }
                    frame "Getriebe & Reifen", Default {
                    }
                  }
                  n145 = call "Verstrichene Zeit"("Time Target (s)"=w684, "Reset"=w685) -> ("Time has Elapsed"=w682:bool)  [unwired: 10 in, 7 out]
                  n146 = case shown="True" w682 {
                    frame False {
                    }
                    frame True {
                      n147 = property on="Untersetzung\nermittelt" class="Bool. (strikt)"("Blinking"=FALSE ("Blinkend"), "BoolText.Text"="Go" ("Boolescher Text.Text")) -> ()  [unwired: 2 in, 2 out]
                    }
                  }
                  "Untersetzung-Graph" <- w686
                }
                frame True {
                }
              }
              n148 = Array Size "Array-Größe"(array=w591) -> (size(s)=w633:i32)
              n149 = Square(x=w607) -> (x^2=w631:dbl)
              n150 = Multiply(x=w591, y=w607) -> (x*y=w613:dbl[])
              n151 = Multiply(x=w613, y=w632) -> (x*y=w628:dbl[])
              n152 = Greater?(x=w633, y=w589) -> (0:w634:bool)
              n153 = Divide(x="Rollenträgheit [kgm²]", y=w631) -> (x/y=w619:dbl)
              n154 = Multiply(x=w619, y=w618) -> (x*y=w617:dbl)
              n155 = And(x=w635, y=w634) -> (x .and. y?=w598:bool)
              n156 = Array Size "Array-Größe"(array=w628) -> (size(s)=w616:i32)
              n157 = Decrement(x=w616) -> (x-1=w615:i32)
              n158 = Select(t=w600, s=w598, f=1000000.0) -> (s? t:f=w601:dbl)
              n159 = Initialize Array(0.0 ("y"), 0) -> (w622:dbl[])
              n160 = for {
                N: w616 -> [_]
                tunnel: "Differenzenquotient" -> [w657]
                tunnel: w628 -> [w665]
                tunnel: w615 -> [w656]
                tunnel: w625 -> [w666]
                shift-right: [w662] -> w614
                shift-left: w622 -> [w663]
                tunnel: w613 -> [w660] mode=indexing
                tunnel: w612 -> [w648]
                tunnel: w601 -> [w659]
                tunnel: [w649] -> w611
                tunnel: w610 -> [w646]
                i -> [w650]
                stop <- w647 stop-if-true
                n161 = Subtract(x=w656, y=w657) -> (x-y=w658:i32)
                n162 = Add(x=w650, y=w657) -> (x+y=w673:i32)
                n163 = Subtract(x=w650, y=w657) -> (x-y=w679:i32)
                n164 = Greater Or Equal?(x=w650, y=w657) -> (x >= y?=w653:bool)
                n165 = Greater?(x=w660, y=w659) -> (0:w661:bool)
                n166 = Max & Min(x=w656, y=w673) -> (min(x,y)=w674:i32)  [unwired: 1 out]
                n167 = Max & Min(x=w679, y=0) -> (max(x,y)=w677:i32)  [unwired: 1 out]
                n168 = Subtract(x=w674, y=w650) -> (x-y=w675:i32)
                n169 = Subtract(x=w650, y=w677) -> (x-y=w676:i32)
                n170 = Less Or Equal?(x=w650, y=w658) -> (x <= y?=w654:bool)
                n171 = Max & Min(x=w676, y=w675) -> (min(x,y)=w667:i32)  [unwired: 1 out]
                n172 = Add(x=w650, y=w667) -> (x+y=w672:i32)
                n173 = Subtract(x=w650, y=w667) -> (x-y=w671:i32)
                n174 = Multiply(x=w667, y=w666) -> (x*y=w664:dbl)
                n175 = Index Array(array=w665, index=w672) -> (element=w669:dbl)
                n176 = Index Array(array=w665, index=w671) -> (element=w670:dbl)
                n177 = Subtract(x=w669, y=w670) -> (x-y=w668:dbl)
                n178 = Divide(x=w668, y=w664) -> (x/y=w655:dbl)
                n179 = Less Than 0?(x=w655) -> (x < 0?=w652:bool)
                n180 = Less Or Equal To 0?(x=w648) -> (x <= 0?=w651:bool)
                n181 = Build Array (concatenate)(w663, w655) -> (w662:dbl[])
                n182 = Compound Arithmetic op=AND(w652, w661, w651, w653, w654, w646) -> (w647:bool)
                n183 = case shown="True" w647 {
                  tunnel: w650 -> [_ w681]
                  tunnel: [w680 w681] -> w649
                  tunnel: w648 -> [w680 _]
                  frame False {
                  }
                  frame True {
                  }
                }
              }
              n184 = Multiply(x=w614, y=w617) -> (x*y=w630:dbl[])
              n185 = Multiply(x=w628, y=w630) -> (x*y=w620:dbl[])
              n186 = Multiply(x=w621, y=w620) -> (x*y=w629:dbl[])
            }
          }
          "Untersetzung\nermittelt" <- w512
          n187 = local read "Start"() -> (w458:bool)
          n188 = Greater Than 0?(x=w490) -> (x > 0?=w491:bool)
          n189 = Not(x=w458) -> (.not. x?=w457:bool)
          n190 = Select(t=w511, s=w512, f=0.0) -> (s? t:f=→"Untersetzung":dbl)
          n191 = Or(x=w491, y=w457) -> (x .or. y?=w494:bool)
        }
        n192 = VISA Clear(VISA resource name=w6, error in (no error)=w5) -> (VISA resource name out=w3:refnum<visa-resource-name>, error out=w7:errorcluster)
        n193 = VISA Close(VISA resource name=w3, error in (no error)=w7) -> ()  [unwired: 1 out]
        n194 = case shown="True" w39 {
          tunnel: w37 -> [_ w428]
          tunnel: w36 -> [_ w433]
          tunnel: w35 -> [_ w432]
          tunnel: w34 -> [_ w404]
          tunnel: w33 -> [_ w429]
          tunnel: w32 -> [_ w427]
          tunnel: w31 -> [_ w421]
          tunnel: w26 -> [_ w407]
          tunnel: ["" w406] -> w27
          tunnel: w28 -> [_ w405]
          tunnel: ["" w403] -> _
          tunnel: [w367 w380] -> w24
          tunnel: [w367 w379] -> w23
          tunnel: [w367 w378] -> w22
          frame False {
            w368 = 0.0
            n195 = Initialize Array(w368, w368) -> (w367:dbl[])
          }
          frame True {
            w392 = 735.498  # PS in W
            w398 = 0.10471975511965978  # w = (2 * Pi / 60) * n
            w402 = 0
            n196 = Array Subset "P"(array=w432, length=w404) -> (w424:dbl[])  [unwired: 1 in]
            n197 = Array Subset "M"(array=w433, length=w404) -> (w425:dbl[])  [unwired: 1 in]
            n198 = Array Subset "alpha"(array=w429, length=w404) -> (w430:dbl[])  [unwired: 1 in]
            n199 = Array Subset "n"(array=w428, length=w404) -> (w426:dbl[])  [unwired: 1 in]
            n200 = property on="Pmax" class="Str"("Text.FontSize"=48) -> ()  [unwired: 2 in, 2 out]
            n201 = property on="Ergebnis" class="Str"("Text.FontSize"=18) -> ()  [unwired: 2 in, 2 out]
            n202 = Array Size(array=w430) -> (size(s)=w431:i32)
            n203 = for {
              N: w431 -> [w451]
              tunnel: w429 -> [w448]
              tunnel: w428 -> [w445]
              tunnel: w427 -> [w442]
              tunnel: [w440] -> w400
              i -> [w446]
              stop <- w441 stop-if-true
              n204 = Decrement(x=w451) -> (x-1=w450:i32)
              n205 = Subtract(x=w450, y=w446) -> (x-y=w440:i32)
              n206 = Index Array(array=w448, index=w440) -> (element=w449:dbl)
              n207 = Index Array(array=w445, index=w440) -> (element=w444:dbl)
              n208 = Less?(x=w444, y=w442) -> (x < y?=w443:bool)
              n209 = Less Or Equal To 0?(x=w449) -> (x <= 0?=w447:bool)
              n210 = And(x=w447, y=w443) -> (x .and. y?=w441:bool)
            }
            n211 = Increment(x=w400) -> (x+1=w399:i32)
            n212 = Array Subset "P"(array=w424, index=w399) -> (w401:dbl[])  [unwired: 1 in]
            n213 = Array Subset "M"(array=w425, index=w399) -> (w397:dbl[])  [unwired: 1 in]
            n214 = Array Subset "n"(array=w426, index=w399) -> (w380:dbl[])  [unwired: 1 in]
            n215 = Array Max & Min "nmax [1/min]"(array=w380) -> (max value=w423:dbl)  [unwired: 3 out]
            n216 = local write "Polynom"("Polynom") -> ()
            n217 = Bundle(w380, w401) -> (w384:cluster{dbl[], dbl[]})  [unwired: 1 in]
            n218 = Bundle(w380, w397) -> (w385:cluster{dbl[], dbl[]})  [unwired: 1 in]
            n219 = Multiply(x=w380, y=w398) -> (x*y=w394:dbl[])
            n220 = Array Size(array=w380) -> (size(s)=w377:i32)
            n221 = call <vilib>:"General Polynomial Fit.vi"("Y"=w397, "polynomial order"="Polynom", "X"=w380, "method"=T4."Biquadrat" ("Methode"), "algorithm"=3) -> ("Best Polynomial Fit"=w379:dbl[])  [unwired: 7 in, 3 out]
            n222 = Bundle(w380, "Best Polynomial Fit"=w379) -> (w386:cluster{dbl[], "Best Polynomial Fit":dbl[]})  [unwired: 1 in]
            n223 = Multiply(x=w379, y=w394) -> (x*y=w393:dbl[])
            n224 = Multiply(x=w377, y=0.1) -> (x*y=w371:dbl)
            n225 = Multiply(x=w377, y=0.8) -> (x*y=w388:dbl)
            n226 = Array Subset "MPoly ohne die ersten\nund letzten paar %"(array=w379, index=w371, length=w388) -> (w382:dbl[])
            n227 = Array Subset "n ohne die ersten \nund letzten paar %"(array=w380, index=w371, length=w388) -> ()  [unwired: 1 out]
            n228 = Divide(x=w423, y=w405) -> (x/y=w422:dbl)
            n229 = Divide(x=w393, y=w392) -> (x/y=w378:dbl[])
            n230 = Array Subset "PPoly ohne die ersten\nund letzten paar %"(array=w378, index=w371, length=w388) -> (w383:dbl[])
            n231 = Bundle(w380, w378) -> (w387:cluster{dbl[], dbl[]})  [unwired: 1 in]
            n232 = Compound Arithmetic op=MULTIPLY "vmax"(w422, w421, 0.06) -> (w413:dbl)
            n233 = Array Max & Min "Mmax"(array=w382) -> (max value=w390:dbl, max index (indices)=w373:i32)  [unwired: 2 out]
            n234 = Add(x=w371, y=w373) -> (x+y=w372:dbl)
            n235 = Multiply(x=w390, y=1.8) -> (x*y=w434:dbl)
            n236 = Index Array "n(Mmax)"(array=w380, index=w372) -> (element=w414:dbl)
            n237 = Array Max & Min "Pmax"(array=w383) -> (max value=w391:dbl, max index (indices)=w375:i32)  [unwired: 2 out]
            n238 = Build Array(w387, w386, w384, w385) -> (→"XY-Graph":cluster{dbl[], "Best Polynomial Fit":dbl[]}[])
            n239 = Add(x=w371, y=w375) -> (x+y=w374:dbl)
            n240 = local read "Luftfeuchtigkeit [%]"() -> (w417:dbl)
            n241 = local read "Lufttemperatur [°C]"() -> (w416:dbl)
            n242 = local read "Luftdruck [mbar]"() -> (w418:dbl)
            n243 = Multiply(x=w391, y=1.2) -> (x*y=w435:dbl)
            n244 = property on="XY-Graph" class="XYGraph (strikt)"("ActYScl"=1, "YScale.Maximum"=w434, "YScale.Minimum"=w402) -> ()  [unwired: 2 in, 2 out]
            n245 = property on="XY-Graph" class="XYGraph (strikt)"("ActYScl"=w402, "YScale.Maximum"=w435, "YScale.Minimum"=w402) -> ()  [unwired: 2 in, 2 out]
            n246 = Index Array "n(Pmax)"(array=w380, index=w374) -> (element=w419:dbl)
            n247 = Format Into String(format string="%.1f PS" ("Format-String"), w391) -> (resulting string=→"Pmax":string)  [unwired: 2 in, 1 out]
            n248 = Format Date/Time String(time format string (%c)="%x %H:%M ") -> (date/time string=w406:string)  [unwired: 2 in]
            n249 = Format Into String(format string="%.1f PS bei %d 1/min   |   %.1f Nm bei %d 1/min   |   vmax: %d km/h\\nDIN 70020 k =%.3f (%d \\B0C, %d %%, %d mbar)\\n%s" ("Format-String"), w391, w419, w390, w414, w413, w407, w416, w417, w418, w406) -> (resulting string=w403:string)  [unwired: 2 in, 1 out]
            "Ergebnis" <- w403
          }
        }
        n250 = flat-sequence {
          tunnel: w16 -> [w325]
          tunnel: w18 -> [w326]
          tunnel: w22 -> [w327]
          tunnel: w23 -> [w328]
          tunnel: w24 -> [w329]
          tunnel: w25 -> [w330]
          tunnel: w26 -> [w331]
          tunnel: w27 -> [w332]
          tunnel: w28 -> [w333]
          tunnel: w29 -> [w334]
          tunnel: w30 -> [w335]
          tunnel: [w335] -> w129
          tunnel: [w334] -> w128
          tunnel: [w333] -> w127
          tunnel: [w332] -> w126
          tunnel: [w331] -> w125
          tunnel: [w330] -> w124
          tunnel: [w329] -> w123
          tunnel: [w328] -> w122
          tunnel: [w327] -> w121
          tunnel: [w326] -> w120
          tunnel: [w325] -> w119
          tunnel: [w321] -> w4
          tunnel: w3 -> [w321]
          tunnel: w129 -> [w366]
          tunnel: w128 -> [w365]
          tunnel: w127 -> [w364]
          tunnel: w126 -> [w363]
          tunnel: w125 -> [w362]
          tunnel: w124 -> [w361]
          tunnel: w123 -> [w360]
          tunnel: w122 -> [w359]
          tunnel: w121 -> [w358]
          tunnel: w120 -> [w357]
          tunnel: w119 -> [w356]
          tunnel: w4 -> [w337]
          frame #0 {
            w323 = FALSE ("Start [F1]")
            w324 = 0  # Aktivieren
            n251 = local write "Start"(w323) -> ()
            n252 = property on="Speichern" class="Bool. (strikt)"("DisabledEnum"=w324) -> ()  [unwired: 2 in, 2 out]
            n253 = property on="Übersetzung ermitteln aus" class="Enum (strikt)"("DisabledEnum"=w324) -> ()  [unwired: 2 in, 2 out]
            n254 = property on="Konfiguration:" class="Bool. (strikt)"("DisabledEnum"=w324) -> ()  [unwired: 2 in, 2 out]
            n255 = property on="Ende" class="Bool. (strikt)"("DisabledEnum"=w324) -> ()  [unwired: 2 in, 2 out]
            n256 = property on="Drucken" class="Bool. (strikt)"("DisabledEnum"=w324) -> ()  [unwired: 2 in, 2 out]
            n257 = property on="Untersetzung\nermittelt" class="Bool. (strikt)"("BoolText.Text"="GO" ("Boolescher Text.Text"), "Blinking"=w323) -> ()  [unwired: 2 in, 2 out]
            n258 = local write "Untersetzung\nermittelt"(w323) -> ()
          }
          frame #1 {
            w340 = 0.0
            n259 = local read "Übersetzung ermitteln aus"() -> (w343:T2)
            n260 = local read "Rollenträgheit [kgm²]"() -> (w353:dbl)
            n261 = local read "Gleitender Mittelwert"() -> (w349:u8)
            n262 = local read "Messung Klimadaten"() -> (w339:bool)
            n263 = local read "Rollengeber [Inkr/U]"() -> (w354:u16)
            n264 = local read "Differenzenquotient"() -> (w348:u8)
            n265 = local read "Lufttemperatur [°C]"() -> (w346:dbl)
            n266 = local read "Luftfeuchtigkeit [%]"() -> (w345:dbl)
            n267 = local read "Reifenumfang [m]"() -> (w350:dbl)
            n268 = local read "n vom Gas [1/min]"() -> (w341:dbl)
            n269 = local read "Zündung [Imp/U]"() -> (w352:dbl)
            n270 = local read "Luftdruck [mbar]"() -> (w344:dbl)
            n271 = local read "nKuWe/nRolle"() -> (w336:dbl)
            n272 = local read "Getriebe [1:]"() -> (w351:dbl)
            n273 = local read "Polynom"() -> (w347:u8)
            n274 = local read "Dauer [s]"() -> (w342:dbl)
            n275 = Bundle("Fahrzeugdaten"="Fahrzeugdaten", "date/time string"=w363, "Rollengeber [Inkr/U]"=w354, "Rollenumfang [m]"=w361, "Rollenträgheit [kgm²]"=w353, "Zündung [Imp/U]"=w352, "Getriebe [1:]"=w351, "Reifenumfang [m]"=w350, "mean value"=w364, "Gleitender Mittelwert"=w349, "Differenzenquotient"=w348, "Polynom"=w347, w366, "element"=w362, "Lufttemperatur [°C]"=w346, "Luftfeuchtigkeit [%]"=w345, "Luftdruck [mbar]"=w344, w365, w360, "Best Polynomial Fit"=w359, w358, "Übersetzung ermitteln aus"=w343, "Dauer [s]"=w342, w340, w340, "n vom Gas [1/min]"=w341, w357, w356, "Messung Klimadaten"=w339, "VISA resource name out"=w337, "nKuWe/nRolle"=w336) -> (→"Datenspeicher":T6)  [unwired: 1 in]
          }
        }
      }
    }
    n276 = local read "Ende"() -> (w1:bool)
  }
  n277 = flat-sequence {
    frame #0 {
      n278 = call <vilib>:"Application Directory.vi"() -> ("Application Directory"=w824:path)
      n279 = Build Path(base path=w824, name or relative path="Konfig.xml") -> (appended path=w822:path)
      n280 = call-poly <vilib>:"Read From XML File.vi"("XML File Path"=w822) -> ("error out"=w803:errorcluster, "XML Elements"=w826:string)  [unwired: 8 in, 1 out]
      n281 = property on="Datenspeicher" class="Cluster (strikt)"() -> ("Value"=w825:T3)  [unwired: 2 in, 2 out]
      n282 = case shown="Kein Fehler" w803 {
        tunnel: w826 -> [w829 _]
        tunnel: w825 -> [w828 _]
        tunnel: [w827 T7 {"Fahrzeugdaten"="", "date/time string"="05.02.2017 22:14 ", "Rolle [Inkr/U]"=10, "Rollenumfang [m]"=0.613, "Rollenträgheit [kgm²]"=0.402, "Zündung [Imp/U]"=5.0, "Getriebe [1:]"=5.343, "Reifenumfang [m] "=1.222, "element"=2.0, "Gl. Mittelwert"=35, "Differenzenquotient"=12, "Polynom"=15, "element"=0.01639344262295082, "element"=1.0177230216140456, "Lufttemperatur [°C]"=23.3, "Luftfeuchtigkeit [%]"=43.8, "Luftdruck [mbar]"=1013.45, array[1238 elements], array[1224 elements], "Best Polynomial Fit"=array[1224 elements], array[1224 elements], "Übersetzung ermitteln aus"=0, "[s]"=5.0, "nmin [1/min]"=0.0, "nmax [1/min]"=0.0, "n vom Gas [1/min]"=5000.0, array[1238 elements], array[1238 elements], "Boolesch"=TRUE, "Serielle Schnittstelle"="", 10.0} ("Datenspeicher")] -> w804
        frame No Error {
          n283 = Unflatten From XML(xml string=w829, type=w828) -> (value=w827:T3)  [unwired: 1 in, 1 out]
        }
        frame Error {
        }
      }
      n284 = property on="Datenspeicher" class="Cluster (strikt)"("Value"=w804) -> ()  [unwired: 2 in, 2 out]
      n285 = Unbundle(w804) -> ("Fahrzeugdaten"=w821:string, "Rolle [Inkr/U]"=w820:u16, "Rollenumfang [m]"=w819:dbl, "Rollenträgheit [kgm²]"=w818:dbl, "Zündung [Imp/U]"=w817:dbl, "Getriebe [1:]"=w816:dbl, "Reifenumfang [m]"=w815:dbl, "element"=w802:dbl, "Gl. Mittelwert"=w814:u8, "Differenzenquotient"=w813:u8, "Polynom"=w812:u8, "Lufttemperatur [°C]"=w811:dbl, "Luftfeuchtigkeit [%]"=w810:dbl, "Luftdruck [mbar]"=w809:dbl, "Übersetzung ermitteln aus"=w806:u8, "[s]"=w808:dbl, "n vom Gas [1/min]"=w807:dbl, "Boolesch"=w805:bool, "Serielle Schnittstelle"=w801:refnum<visa-resource-name>, "nKuWe/nRolle"=w800:dbl)  [unwired: 11 out]
      n286 = property on="Polynom" class="DigWert (strikt)"("Value"=w812) -> ()  [unwired: 2 in, 2 out]
      n287 = property on="Dauer [s]" class="DigWert (strikt)"("Value"=w808) -> ()  [unwired: 2 in, 2 out]
      n288 = property on="Fahrzeugdaten" class="Str"("Value"=w821) -> ()  [unwired: 2 in, 2 out]
      n289 = property on="Rollengeber [Inkr/U]" class="DigWert (strikt)"("Value"=w820) -> ()  [unwired: 2 in, 2 out]
      n290 = property on="Rollenumfang [m]" class="DigWert (strikt)"("Value"=w819) -> ()  [unwired: 2 in, 2 out]
      n291 = property on="Rollenträgheit [kgm²]" class="DigWert (strikt)"("Value"=w818) -> ()  [unwired: 2 in, 2 out]
      n292 = property on="Zündung [Imp/U]" class="DigWert (strikt)"("Value"=w817) -> ()  [unwired: 2 in, 2 out]
      n293 = property on="Getriebe [1:]" class="DigWert (strikt)"("Value"=w816) -> ()  [unwired: 2 in, 2 out]
      n294 = property on="Reifenumfang [m]" class="DigWert (strikt)"("Value"=w815) -> ()  [unwired: 2 in, 2 out]
      n295 = property on="nKuWe/nRolle" class="DigWert (strikt)"("Value"=w802) -> ()  [unwired: 2 in, 2 out]
      n296 = property on="Gleitender Mittelwert" class="DigWert (strikt)"("Value"=w814) -> ()  [unwired: 2 in, 2 out]
      n297 = property on="Differenzenquotient" class="DigWert (strikt)"("Value"=w813) -> ()  [unwired: 2 in, 2 out]
      n298 = property on="Lufttemperatur [°C]" class="DigWert (strikt)"("Value"=w811) -> ()  [unwired: 2 in, 2 out]
      n299 = property on="Luftfeuchtigkeit [%]" class="DigWert (strikt)"("Value"=w810) -> ()  [unwired: 2 in, 2 out]
      n300 = property on="Luftdruck [mbar]" class="DigWert (strikt)"("Value"=w809) -> ()  [unwired: 2 in, 2 out]
      n301 = property on="Übersetzung ermitteln aus" class="Enum (strikt)"("Val(Sgnl)"=w806) -> ()  [unwired: 2 in, 2 out]
      n302 = property on="n vom Gas [1/min]" class="DigWert (strikt)"("Value"=w807) -> ()  [unwired: 2 in, 2 out]
      n303 = property on="Messung Klimadaten" class="Bool. (strikt)"("Val(Sgnl)"=w805) -> ()  [unwired: 2 in, 2 out]
      n304 = local write "Serielle Schnittstelle"(w801) -> ()
      n305 = property on="nKuWe/nRolle" class="DigWert (strikt)"("Value"=w800) -> ()  [unwired: 2 in, 2 out]
    }
    frame #1 {
      w837 = 2  # Deaktivieren
      w839 = 0.0  # Graphen löschen
      n306 = local read "Serielle Schnittstelle"() -> (w835:refnum<visa-resource-name>)
      n307 = property on="Frontpanel-Position" class="Bereich"("Origin"=T8 {"Horizontal"=8, "Vertical"=6}) -> ()  [unwired: 2 in, 2 out]
      n308 = property on="Füllstand Lesepuffer" class="Schieber (strikt)"("Scale.Maximum"=100) -> ()  [unwired: 2 in, 2 out]
      n309 = property on="Drucken" class="Bool. (strikt)"("DisabledEnum"=w837) -> ()  [unwired: 2 in, 2 out]
      n310 = property on="Speichern" class="Bool. (strikt)"("DisabledEnum"=w837) -> ()  [unwired: 2 in, 2 out]
      n311 = Build Array(w839) -> (w838:dbl[])
      n312 = VISA Clear(VISA resource name=w835) -> (VISA resource name out=w834:refnum<visa-resource-name>, error out=w833:errorcluster)  [unwired: 1 in]
      n313 = property on="Untersetzung-Graph" class="SVDiagr (strikt)"("History Data"=w838) -> ()  [unwired: 2 in, 2 out]
      n314 = VISA Close(VISA resource name=w834, error in (no error)=w833) -> (error out=w832:errorcluster)
      n315 = case shown="Kein Fehler" w832 {
        tunnel: [T5."Enabled" ("Deaktiviert") T5."Disabled and Grayed Out" ("Deaktiviert")] -> w831
        frame No Error {
        }
        frame Error {
        }
      }
      n316 = property on="Start" class="Bool. (strikt)"("DisabledEnum"=w831) -> ()  [unwired: 2 in, 2 out]
    }
  }
  n317 = while {
    stop <- w843 stop-if-true
    n318 = event shown="[0] \"Konfiguration:\": Wertänderung" {
      selector: _ -> [_ _ _ _ _ _ _ _]
      dyn-events: _ -> [_ _ _ _ _ _ _ _]
      timeout: _ -> [_ _ _ _ _ _ _ _]
      tunnel: [_ _ _ TRUE _ _ _ _] -> w843
      event "Konfiguration:": Value Change {
        n319 = event-data() -> ("OldVal"=w845:bool)  [unwired: 1 in, 5 out]
        n320 = flat-sequence {
          tunnel: [w849] -> w846
          tunnel: w845 -> [w849]
          tunnel: w846 -> [w876]
          frame #0 {
            n321 = call-poly <vilib>:"Read From XML File.vi"() -> ("error out"=w847:errorcluster, "XML Elements"=w850:string)  [unwired: 9 in, 1 out]
            n322 = property on="Datenspeicher" class="Cluster (strikt)"() -> ("Value"=w848:T3)  [unwired: 2 in, 2 out]
            n323 = case shown="Kein Fehler" w847 {
              selector: w847 -> [_ w875]
              tunnel: w850 -> [w854 _]
              tunnel: w848 -> [w853 _]
              frame No Error {
                n324 = Unflatten From XML(xml string=w854, type=w853) -> (value=w852:T3, error out=w851:errorcluster)  [unwired: 1 in]
                n325 = case shown="Kein Fehler" w851 {
                  tunnel: w852 -> [w873 _]
                  frame No Error {
                    n326 = Unbundle(w873) -> ("Fahrzeugdaten"=w872:string, "Rolle [Inkr/U]"=w871:u16, "Rollenumfang [m]"=w870:dbl, "Rollenträgheit [kgm²]"=w869:dbl, "Zündung [Imp/U]"=w868:dbl, "Getriebe [1:]"=w867:dbl, "Reifenumfang [m]"=w866:dbl, "Gl. Mittelwert"=w865:u8, "Differenzenquotient"=w864:u8, "Polynom"=w863:u8, "Lufttemperatur [°C]"=w862:dbl, "Luftfeuchtigkeit [%]"=w861:dbl, "Luftdruck [mbar]"=w860:dbl, "Übersetzung ermitteln aus"=w857:u8, "[s]"=w859:dbl, "n vom Gas [1/min]"=w858:dbl, "Boolesch"=w856:bool, "nKuWe/nRolle"=w855:dbl)  [unwired: 13 out]
                    n327 = property on="Polynom" class="DigWert (strikt)"("Value"=w863) -> ()  [unwired: 2 in, 2 out]
                    n328 = property on="Dauer [s]" class="DigWert (strikt)"("Value"=w859) -> ()  [unwired: 2 in, 2 out]
                    n329 = property on="Fahrzeugdaten" class="Str"("Value"=w872) -> ()  [unwired: 2 in, 2 out]
                    n330 = property on="Rollengeber [Inkr/U]" class="DigWert (strikt)"("Value"=w871) -> ()  [unwired: 2 in, 2 out]
                    n331 = property on="Rollenumfang [m]" class="DigWert (strikt)"("Value"=w870) -> ()  [unwired: 2 in, 2 out]
                    n332 = property on="Rollenträgheit [kgm²]" class="DigWert (strikt)"("Value"=w869) -> ()  [unwired: 2 in, 2 out]
                    n333 = property on="Zündung [Imp/U]" class="DigWert (strikt)"("Value"=w868) -> ()  [unwired: 2 in, 2 out]
                    n334 = property on="Getriebe [1:]" class="DigWert (strikt)"("Value"=w867) -> ()  [unwired: 2 in, 2 out]
                    n335 = property on="Reifenumfang [m]" class="DigWert (strikt)"("Value"=w866) -> ()  [unwired: 2 in, 2 out]
                    n336 = property on="Gleitender Mittelwert" class="DigWert (strikt)"("Value"=w865) -> ()  [unwired: 2 in, 2 out]
                    n337 = property on="Differenzenquotient" class="DigWert (strikt)"("Value"=w864) -> ()  [unwired: 2 in, 2 out]
                    n338 = property on="Lufttemperatur [°C]" class="DigWert (strikt)"("Value"=w862) -> ()  [unwired: 2 in, 2 out]
                    n339 = property on="Luftfeuchtigkeit [%]" class="DigWert (strikt)"("Value"=w861) -> ()  [unwired: 2 in, 2 out]
                    n340 = property on="Luftdruck [mbar]" class="DigWert (strikt)"("Value"=w860) -> ()  [unwired: 2 in, 2 out]
                    n341 = property on="Übersetzung ermitteln aus" class="Enum (strikt)"("Val(Sgnl)"=w857) -> ()  [unwired: 2 in, 2 out]
                    n342 = property on="n vom Gas [1/min]" class="DigWert (strikt)"("Value"=w858) -> ()  [unwired: 2 in, 2 out]
                    n343 = property on="Messung Klimadaten" class="Bool. (strikt)"("Val(Sgnl)"=w856) -> ()  [unwired: 2 in, 2 out]
                    n344 = property on="nKuWe/nRolle" class="DigWert (strikt)"("Value"=w855) -> ()  [unwired: 2 in, 2 out]
                  }
                  frame Error {
                    n345 = One Button Dialog(message="Dateiversion nicht kompatibel" ("Nachricht")) -> ()  [unwired: 1 in, 1 out]
                  }
                }
              }
              frame Error {
                n346 = call <vilib>:"Clear Errors.vi"("error in (no error)"=w875) -> ()  [unwired: 5 in, 2 out]
              }
            }
          }
          frame #1 {
            n347 = property on="Konfiguration:" class="Bool. (strikt)"("Value"=w876) -> ()  [unwired: 2 in, 2 out]
          }
        }
      }
      event "Drucken": Value Change {
        n348 = event-data() -> ("OldVal"=w877:bool)  [unwired: 1 in, 5 out]
        n349 = flat-sequence {
          tunnel: [w882] -> w878
          tunnel: w877 -> [w882]
          tunnel: w878 -> [w883]
          frame #0 {
            n350 = control-ref of="Fahrzeugdaten"() -> (w880:refnum<vi>)
            n351 = control-ref of="XY-Graph"() -> (w881:refnum<vi>)
            n352 = control-ref of="Ergebnis"() -> (w879:refnum<vi>)
            n353 = call "printgraph_V0.01.vi"("reference 2"=w879, "Fahrzeugdaten"=w880, "XYGraph (Eingang)"=w881) -> ()  [unwired: 9 in]
          }
          frame #1 {
            n354 = property on="Drucken" class="Bool. (strikt)"("Value"=w883) -> ()  [unwired: 2 in, 2 out]
          }
        }
      }
      event "Speichern": Value Change {
        n355 = event-data() -> ("OldVal"=w885:bool)  [unwired: 1 in, 5 out]
        n356 = control-ref of="Datenspeicher"() -> (w884:refnum<vi>)
        n357 = local write "Speichern"(w885) -> ()
        n358 = call "savecluster_V0.01.vi"("Datenspeicher 3"=w884) -> ()  [unwired: 2 in]
      }
      event "Ende": Value Change {
        w887 = 0.0 ("element")
        (unwired) 0.0 ("element")
        n359 = event-data() -> ("OldVal"=w917:bool)  [unwired: 1 in, 5 out]
        n360 = local write "Ende"(w917) -> ()
        n361 = local read "Datenspeicher"() -> (w888:T3)
        n362 = Unbundle By Name(w888) -> ("Rolle [Inkr/U]"=w909:u16, "Rollenumfang [m]"=w908:dbl, "Rollenträgheit [kgm²]"=w907:dbl, "Zündung [Imp/U]"=w906:dbl, "Getriebe [1:]"=w905:dbl, "Reifenumfang [m]"=w904:dbl, "Gl. Mittelwert"=w903:u8, "Differenzenquotient"=w902:u8, "Polynom"=w901:u8, "Lufttemperatur [°C]"=w900:dbl, "Luftfeuchtigkeit [%]"=w899:dbl, "Luftdruck [mbar]"=w897:dbl, "Best Polynomial Fit"=w898:dbl[], "Übersetzung ermitteln aus"=w896:u8, "[s]"=w895:dbl, "nmin [1/min]"=w894:dbl, "nmax [1/min]"=w893:dbl, "n vom Gas [1/min]"=w892:dbl, "Boolesch"=w891:bool, "Serielle Schnittstelle"=w886:refnum<visa-resource-name>)  [unwired: 3 out]
        n363 = call <vilib>:"Application Directory.vi"() -> ("Application Directory"=w914:path)
        n364 = Bundle By Name(cluster=w888, "Fahrzeugdaten"="", "date/time string"="", "Rolle [Inkr/U]"=w909, "Rollenumfang [m]"=w908, "Rollenträgheit [kgm²]"=w907, "Zündung [Imp/U]"=w906, "Getriebe [1:]"=w905, "Reifenumfang [m]"=w904, "element"=0.0, "Gl. Mittelwert"=w903, "Differenzenquotient"=w902, "Polynom"=w901, "element"=w887, "element"=w887, "Lufttemperatur [°C]"=w900, "Luftfeuchtigkeit [%]"=w899, "Luftdruck [mbar]"=w897, "Best Polynomial Fit"=w898, "Übersetzung ermitteln aus"=w896, "[s]"=w895, "nmin [1/min]"=w894, "nmax [1/min]"=w893, "n vom Gas [1/min]"=w892, "Boolesch"=w891, "Serielle Schnittstelle"=w886) -> (w889:T3)
        n365 = Build Path(base path=w914, name or relative path="Konfig.xml") -> (appended path=w912:path)
        n366 = Flatten To XML(anything=w889) -> (xml string=w916:string)
        n367 = call-poly <vilib>:"Write to XML File.vi"("XML Input"=w916, "XML File Path"=w912) -> ("error out"=w915:errorcluster)  [unwired: 7 in, 2 out]
        n368 = case shown="Kein Fehler" w915 {
          frame No Error {
          }
          frame Error {
          }
        }
      }
      event "Serielle Schnittstelle": Value Change {
        n369 = event-data() -> ()  [unwired: 1 in, 6 out]
        n370 = property on="Start" class="Bool. (strikt)"("DisabledEnum"=T5."Enabled" ("Deaktiviert")) -> ()  [unwired: 2 in, 2 out]
      }
      event "Messung Klimadaten": Value Change {
        n371 = event-data() -> ("NewVal"=w920:bool)  [unwired: 1 in, 5 out]
        n372 = case shown="True" w920 {
          frame True {
            w921 = T5."Disabled and Grayed Out" ("Deaktiviert")
            n373 = property on="Lufttemperatur [°C]" class="DigWert (strikt)"("DisabledEnum"=w921) -> ()  [unwired: 2 in, 2 out]
            n374 = property on="Luftdruck [mbar]" class="DigWert (strikt)"("DisabledEnum"=w921) -> ()  [unwired: 2 in, 2 out]
            n375 = property on="Luftfeuchtigkeit [%]" class="DigWert (strikt)"("DisabledEnum"=w921) -> ()  [unwired: 2 in, 2 out]
          }
          frame False {
            w922 = T5."Enabled" ("Deaktiviert")
            n376 = property on="Lufttemperatur [°C]" class="DigWert (strikt)"("DisabledEnum"=w922) -> ()  [unwired: 2 in, 2 out]
            n377 = property on="Luftdruck [mbar]" class="DigWert (strikt)"("DisabledEnum"=w922) -> ()  [unwired: 2 in, 2 out]
            n378 = property on="Luftfeuchtigkeit [%]" class="DigWert (strikt)"("DisabledEnum"=w922) -> ()  [unwired: 2 in, 2 out]
          }
        }
      }
      event "Recalc": Value Change {
        n379 = event-data() -> ("OldVal"=w925:bool)  [unwired: 1 in, 5 out]
        n380 = property on="Recalc" class="Bool. (strikt)"("Value"=w925) -> ()  [unwired: 2 in, 2 out]
        n381 = property on="Datenspeicher" class="Cluster (strikt)"() -> ("Value"=w923:T3)  [unwired: 2 in, 2 out]
        n382 = call "ReCalc_V0.16.vi"("Berechnen"=TRUE, "Datenspeicher"=w923) -> ()  [unwired: 3 in]
      }
      event "Übersetzung ermitteln aus": Value Change {
        n383 = event-data() -> ("NewVal"=w927:T2)  [unwired: 1 in, 5 out]
        n384 = case shown="\"nKuWe / nRolle\"" w927 {
          tunnel: [T5."Disabled and Grayed Out" ("Deaktiviert") T5."Disabled and Grayed Out" ("Deaktiviert") T5."Enabled" ("Deaktiviert")] -> w929
          frame "nKuWe / nRolle" {
          }
          frame "Zündsignal", Default {
          }
          frame "Getriebe & Reifen" {
          }
        }
        n385 = case shown="\"Zündsignal\", Standard" w927 {
          tunnel: [T5."Enabled" ("Deaktiviert") T5."Disabled and Grayed Out" ("Deaktiviert") T5."Disabled and Grayed Out" ("Deaktiviert")] -> w928
          frame "nKuWe / nRolle" {
          }
          frame "Zündsignal", Default {
          }
          frame "Getriebe & Reifen" {
          }
        }
        n386 = case shown="\"Zündsignal\", Standard" w927 {
          tunnel: [T5."Disabled and Grayed Out" ("Deaktiviert") T5."Enabled" ("Deaktiviert") T5."Disabled and Grayed Out" ("Deaktiviert")] -> w926
          frame "nKuWe / nRolle" {
          }
          frame "Zündsignal", Default {
          }
          frame "Getriebe & Reifen" {
          }
        }
        n387 = property on="Getriebe [1:]" class="DigWert (strikt)"("DisabledEnum"=w929) -> ()  [unwired: 2 in, 2 out]
        n388 = property on="Reifenumfang [m]" class="DigWert (strikt)"("DisabledEnum"=w929) -> ()  [unwired: 2 in, 2 out]
        n389 = property on="nKuWe/nRolle" class="DigWert (strikt)"("DisabledEnum"=w928) -> ()  [unwired: 2 in, 2 out]
        n390 = property on="Dauer [s]" class="DigWert (strikt)"("DisabledEnum"=w926) -> ()  [unwired: 2 in, 2 out]
        n391 = property on="Zündung [Imp/U]" class="DigWert (strikt)"("DisabledEnum"=w926) -> ()  [unwired: 2 in, 2 out]
      }
    }
    n392 = disable-structure shown="Deaktiviert" {
      disable-tunnel: w843 -> [w844 _]
      frame Disabled {
        n393 = Quit LabVIEW(quit? (T)=w844) -> ()
      }
      frame Enabled {
      }
    }
  }
